vi "N5746A_Initialize.vi"(8 "error":errorcluster, 9 "Reset (T)":bool=TRUE, 10 "ID Query (T)":bool=TRUE, 11 "VISA name":refnum<visa-resource-name>) -> (0 "error out":errorcluster, 3 "VISA out":refnum<visa-resource-name>)   [LabVIEW 2015]
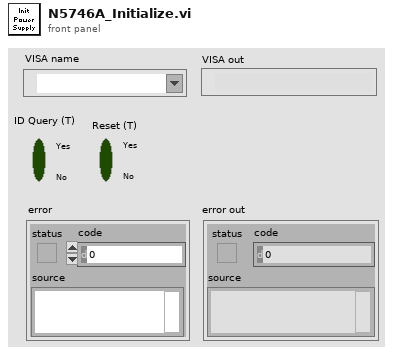
[diagram p1: front panel]
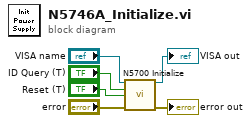
[diagram p0: block diagram]
diagram:
  n1 = call <instrlib>:"N5700 Initialize.vi"("VISA name"="VISA name", "ID Query (T)"="ID Query (T)", "Reset (T)"="Reset (T)", "error in (no error)"="error") -> ("VISA out"=→"VISA out":refnum<visa-resource-name>, "error out"=→"error out":errorcluster)  [unwired: 10 in]
